vi "Take_Snap.vi"(0 "Take Snap \narray":u64[](array[numeric])=[0, 0, 0, 0, 0, 0, 0, 0, 0, 0, 0, 0, 0, 0, 0, 0, 0, 0, 0, 0, 0, 0, 0, 0, 0, 0, 0, 0, 0, 0, 0, 0, 0, 0, 0, 0, 0, 0, 0, 0, 0, 0, 0, 0, 0, 0, 0, 0, 0, 0]) -> (1 "Aborted":bool, 2 "Error Out":u8)   [LabVIEW 2023]
uses:
  <vilib>/rvi/DataTransferAndStorage/Container/XNode/niFpgaContainer.xnode
  <vilib>/rvi/DataTransferAndStorage/Register/Emulation/niFpgaRegisterEmulation.vi
  <vilib>/eio/EIONode/EIONode.xnode
  <vilib>/rvi/eio/common/nirviEmuTemplateMethod_errors.vi
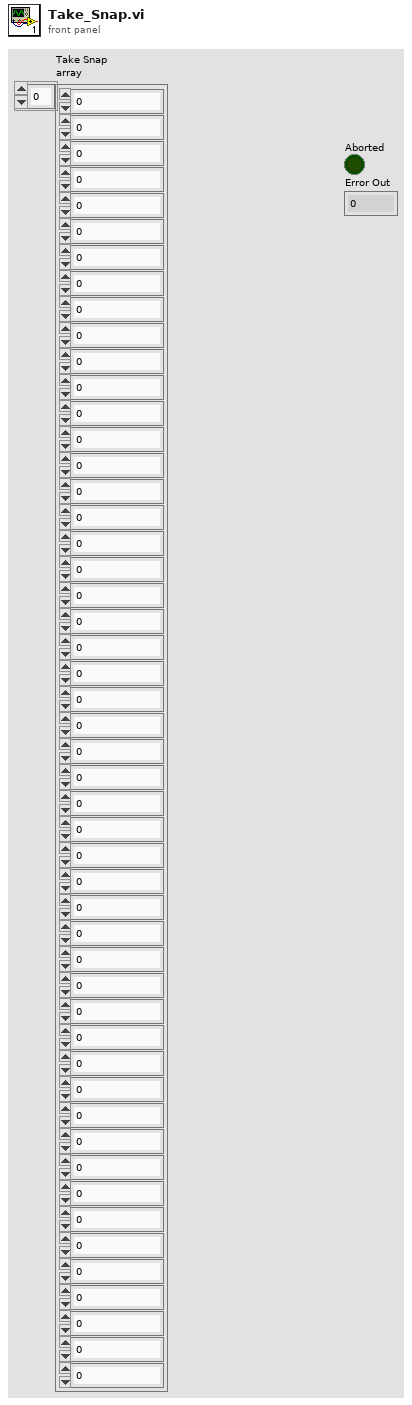
[diagram p1: front panel]
types:
  T1 = cluster{"Boolean array[0]":bool, "Boolean array[1]":bool, "Boolean array[2]":bool, "Boolean array[3]":bool, "Boolean array[4]":bool, "Boolean array[5]":bool, "Boolean array[6]":bool, "Boolean array[7]":bool, "Boolean array[8]":bool, "Boolean array[9]":bool, "Boolean array[10]":bool, "Boolean array[11]":bool, "Boolean array[12]":bool, "Boolean array[13]":bool, "Boolean array[14]":bool, "Boolean array[15]":bool}
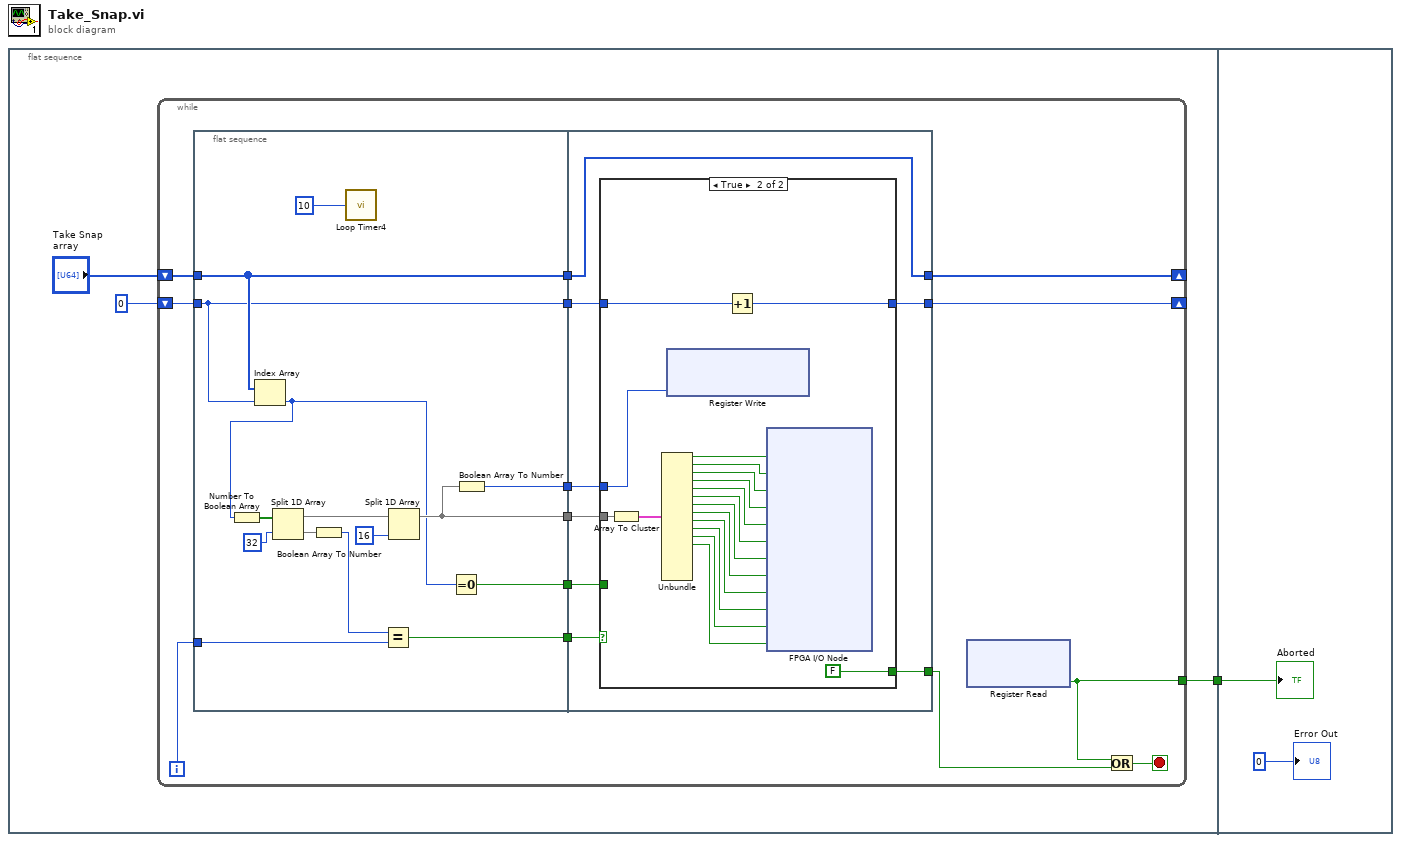
[diagram p0: block diagram]
diagram:
  n1 = flat-sequence {
    tunnel: [w2] -> w1
    tunnel: w1 -> [w63]
    frame #0 {
      n2 = while {
        shift-right: [w8] -> _
        shift-left: i16 0 -> [w11]
        shift-right: [w10] -> _
        shift-left: "Take Snap \narray" -> [w15]
        tunnel: [w5] -> w2
        i -> [w18]
        stop <- w12 stop-if-true
        n3 = flat-sequence {
          tunnel: w18 -> [w27]
          tunnel: [w23] -> w17
          tunnel: [w26] -> w16
          tunnel: w15 -> [w20]
          tunnel: [w24] -> w14
          tunnel: [w22] -> w13
          tunnel: w11 -> [w19]
          tunnel: [w20] -> w9
          tunnel: [w19] -> w7
          tunnel: w17 -> [w41]
          tunnel: w16 -> [w40]
          tunnel: [w39] -> w6
          tunnel: w14 -> [w38]
          tunnel: w13 -> [w37]
          tunnel: [w34] -> w10
          tunnel: w9 -> [w34]
          tunnel: [w36] -> w8
          tunnel: w7 -> [w35]
          frame #0 {
            n4 = Index Array(array=w20, index=w19) -> (element=w21:u64)
            n5 = Number To Boolean Array(number=w21) -> (Boolean array=w31:bool[])
            n6 = Split 1D Array(array=w31, index=32) -> (first subarray=w32:bool[], second subarray=w30:bool[])
            n7 = Boolean Array To Number(Boolean array=w30) -> (number=w25:u32)
            n8 = call "Loop Timer4"("Count(uSec)"=u32 10) -> ()  [unwired: 1 out]
            n9 = Equal?(x=w25, y=w27) -> (x = y?=w26:bool)
            n10 = Split 1D Array(array=w32, index=16) -> (first subarray=w23:bool[])  [unwired: 1 out]
            n11 = Equal To 0?(x=w21) -> (x = 0?=w24:bool)
            n12 = Boolean Array To Number(Boolean array=w23) -> (number=w22:u16)
          }
          frame #1 {
            n13 = case shown="True" w40 {
              tunnel: w41 -> [_ w49]
              tunnel: [w42 FALSE] -> w39
              tunnel: w38 -> [w42 _]
              tunnel: w37 -> [_ w47]
              tunnel: [w43 w45] -> w36
              tunnel: w35 -> [w43 w44]
              frame False {
              }
              frame True {
                n14 = Array To Cluster(array=w49) -> (cluster=w46:T1)
                n15 = Unbundle(w46) -> ("Boolean array[0]"=w61:bool, "Boolean array[1]"=w60:bool, "Boolean array[2]"=w50:bool, "Boolean array[3]"=w51:bool, "Boolean array[4]"=w52:bool, "Boolean array[5]"=w53:bool, "Boolean array[6]"=w54:bool, "Boolean array[7]"=w55:bool, "Boolean array[8]"=w56:bool, "Boolean array[9]"=w57:bool, "Boolean array[10]"=w58:bool, "Boolean array[11]"=w59:bool)  [unwired: 4 out]
                n16 = xnode ("Register Write")("Data"=w47) -> ()  [unwired: 1 in, 1 out]
                n17 = Increment(x=w44) -> (x+1=w45:i16)
                n18 = xnode "FPGA I/O Node"("Mod2/DIO0"=w61, "Mod2/DIO1"=w60, "Mod2/DIO2"=w50, "Mod2/DIO3"=w51, "Mod3/DIO0"=w52, "Mod3/DIO1"=w53, "Mod3/DIO2"=w54, "Mod3/DIO3"=w55, "Mod4/DIO0"=w56, "Mod4/DIO1"=w57, "Mod4/DIO2"=w58, "Mod4/DIO3"=w59) -> ()  [unwired: 12 in, 12 out]
              }
            }
          }
        }
        n19 = xnode ("Register Read")() -> ("Data"=w5:bool)  [unwired: 1 in, 1 out]
        n20 = Or(x=w5, y=w6) -> (x .or. y?=w12:bool)
      }
    }
    frame #1 {
      "Aborted" <- w63
      "Error Out" <- u8 0
    }
  }
